vi "G#Debugger_ListAggregators.vi"(1 "Tree":refnum<vi>, 2 "Aggregator":refnum<vi>, 3 "ObjectIDs":string[](array[string]), 5 "error in (no error)":errorcluster, 6 "AggregatorTags":refnum<vi>) -> (19 "error out":errorcluster)   [LabVIEW 2017, in "G#Debugger.lvlib"]
doc: "Highlights the specified objects in the tree view control."
uses:
  G#Debugger.lvlib
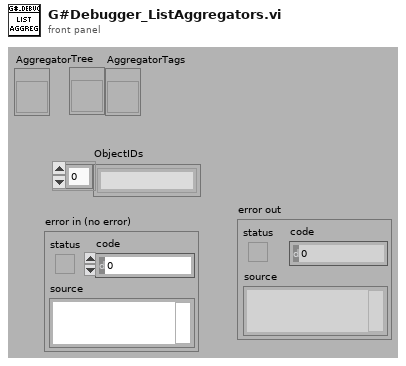
[diagram p1: front panel]
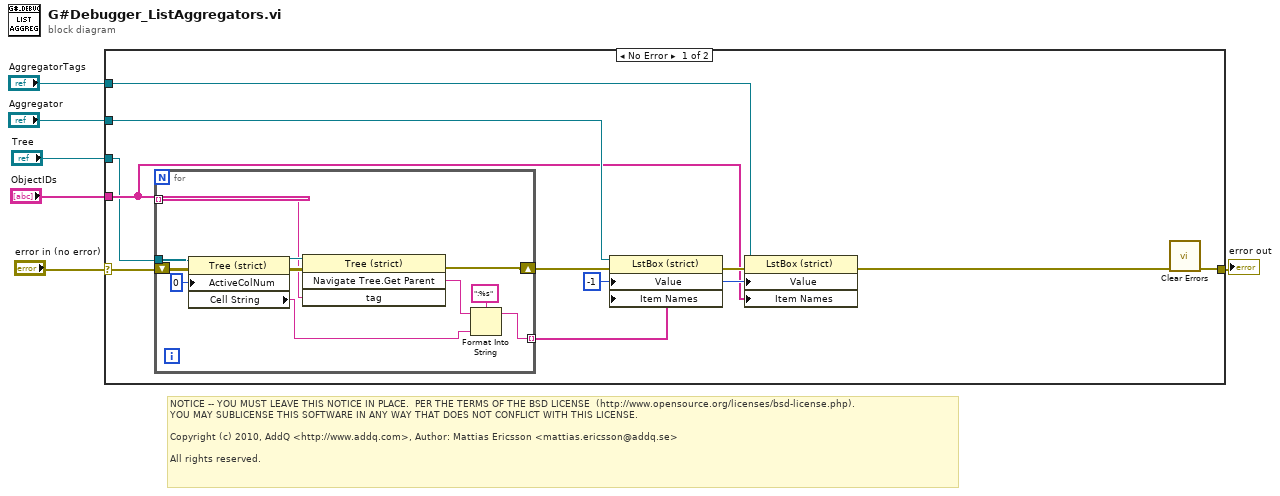
[diagram p0: block diagram]
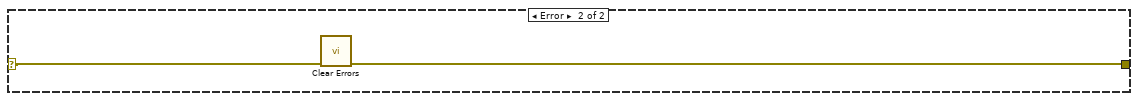
[diagram p2: hidden frame]
diagram:
  # "NOTICE -- YOU MUST LEAVE THIS NOTICE IN PLACE.  PER THE TERMS OF THE BSD LICENSE  (http://www.opensource.org/licenses/bsd-license.php).\nYOU MAY SUBLICENSE THIS SOFTWARE IN ANY WAY THAT DOES NOT CONFLICT WITH THIS LICENSE.\n\nCopyright (c) 2010, AddQ <http://www.addq.com>, Author: Mattias Ericsson <mattias.ericsson@addq.se>\n\nAll rights reserved."
  n1 = case shown="No Error" "error in (no error)" {
    selector: "error in (no error)" -> [w8 w30]
    tunnel: [w17 w29] -> w5
    tunnel: "Tree" -> [w7 _]
    tunnel: "ObjectIDs" -> [w10 _]
    tunnel: "Aggregator" -> [w15 _]
    tunnel: "AggregatorTags" -> [w9 _]
    frame No Error {
      w11 = -1 ("Value")
      n2 = for {
        shift-right: [w25] -> w16
        shift-left: w8 -> [w19]
        tunnel: w10 -> [w24] mode=indexing
        tunnel: w7 -> [w18]
        tunnel: [w20] -> w14 mode=indexing
        n3 = property class="Tree (strict)"(reference=w18, error in=w19, "ActiveColNum"=0 ("Active Cell:Active Column Number")) -> (reference out=w27:refnum<vi>, error out=w26:errorcluster, "Cell String"=w21:string)
        n4 = invoke class="Tree (strict)" method="Navigate Tree.Get Parent"(reference=w27, error in=w26, "tag"=w24) -> (error out=w25:errorcluster, "Navigate Tree:Get Parent"=w23:string)  [unwired: 1 in, 2 out]
        n5 = Format Into String(format string=":%s", initial string=w23, w21) -> (resulting string=w20:string)  [unwired: 1 in, 1 out]
      }
      n6 = property on="Property Node" class="LstBox (strict)"(reference=w15, error in=w16, "Value"=w11, "Item Names"=w14) -> (error out=w13:errorcluster)  [unwired: 1 out]
      n7 = property on="Property Node" class="LstBox (strict)"(reference=w9, error in=w13, "Value"=w11, "Item Names"=w10) -> (error out=w12:errorcluster)  [unwired: 1 out]
      n8 = call <vilib>:"Clear Errors.vi"("error in (no error)"=w12) -> ("error out"=w17:errorcluster)  [unwired: 5 in, 1 out]
    }
    frame Error {
      n9 = call <vilib>:"Clear Errors.vi"("error in (no error)"=w30) -> ("error out"=w29:errorcluster)  [unwired: 5 in, 1 out]
    }
  }
  "error out" <- w5
